vi "ThresholdEstimation(SubVI).vi"(2 "Margin":dbl, 3 "최소값":dbl, 4 "최대값":dbl) -> (0 "N.Th":dbl, 1 "P.Th":dbl)   [LabVIEW 2017]
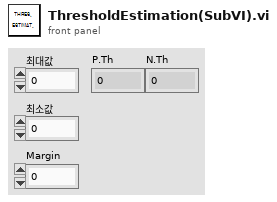
[diagram p1: front panel]
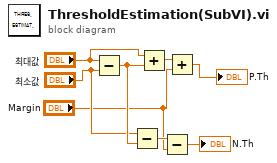
[diagram p0: block diagram]
diagram:
  n1 = Subtract(x="최대값", y="최소값") -> (x-y=w5:dbl)
  n2 = Subtract(x="최소값", y=w5) -> (x-y=w8:dbl)
  n3 = Add(x="최대값", y=w5) -> (x+y=w4:dbl)
  n4 = Subtract(x=w8, y="Margin") -> (x-y=→"N.Th":dbl)
  n5 = Add(x=w4, y="Margin") -> (x+y=→"P.Th":dbl)
